vi "Read All source names.vi"(11 "SolutionBuilder in":refnum<class "SolutionBuilder.lvclass">) -> (2 "All source names":set{string}(c389), 3 "SolutionBuilder out":refnum<class "SolutionBuilder.lvclass">)   [LabVIEW 2019, in "SolutionBuilder.lvlib" / "SolutionBuilder.lvclass"]
uses:
  SolutionBuilder.lvclass
  ProjectItem/ProjectItem.lvclass
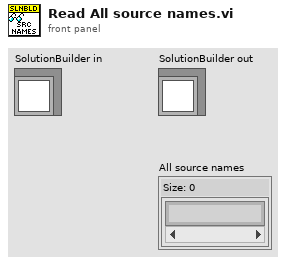
[diagram p1: front panel]
types:
  T1 = typedef "SolutionBuilder.lvlib/SolutionBuilder.lvclass/ProjectItemMap.ctl" = map{path, refnum<class "ProjectItem.lvclass">[]}
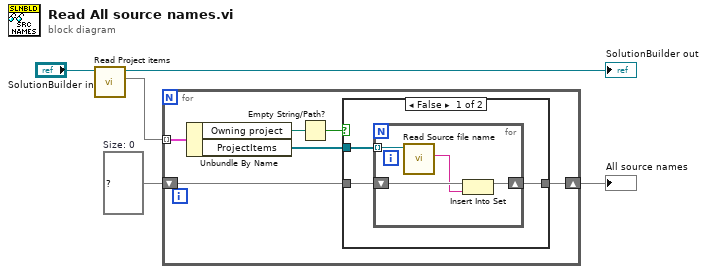
[diagram p0: block diagram]
diagram:
  w5 = set{string} {}  # Size: 0
  n1 = call "Read Project items.vi"("SolutionBuilder in"="SolutionBuilder in") -> ("Project items"=w1:T1, "SolutionBuilder out"=→"SolutionBuilder out":refnum<class "SolutionBuilder.lvclass">)  [unwired: 9 in]
  n2 = for {
    tunnel: w1 -> [w11] mode=indexing
    shift-right: [w7] -> w4
    shift-left: w5 -> [w6]
    n3 = Unbundle By Name(w11) -> ("Owning project"=w10:path, "ProjectItems"=w8:refnum<class "ProjectItem.lvclass">[])
    n4 = Empty String/Path?(string/path=w10) -> (empty?=w9:bool)
    n5 = case shown="False" w9 {
      tunnel: w8 -> [w14 _]
      tunnel: [w13 w19] -> w7
      tunnel: w6 -> [w12 w19]
      frame False {
        n6 = for {
          tunnel: w14 -> [w16] mode=indexing
          shift-right: [w18] -> w13
          shift-left: w12 -> [w17]
          n7 = call "Read Source file name.vi"("ProjectItem in"=w16) -> ("Source file name"=w15:string)  [unwired: 9 in, 1 out]
          n8 = Insert Into Set(10:w15, 11:w17) -> (3:w18:set{string})  [unwired: 1 out]
        }
      }
      frame True {
      }
    }
  }
  "All source names" <- w4
